vi "calibrationElectrometer_getEvent_settingsAppliedReadSets.vi"(8 "error in (no error)":errorcluster, 11 "logevent_settingsAppliedReadSets_Ctl":T1={"avgFilterType"=0, "electId"="                                                                                                                                                                                                                                                                ", "filterActive"=FALSE, "inputRange"=0.0, "integrationTime"=0.0, "medianFilterStatus"=FALSE, "mode"=0, "radingOption"=0, "readingTimeout"=0, "priority"=0}) -> (0 "error out":errorcluster, 2 "function return":i32, 3 "logevent_settingsAppliedReadSets_Ctl out":T1={"avgFilterType"=0, "electId"="                                                                                                                                                                                                                                                                ", "filterActive"=FALSE, "inputRange"=0.0, "integrationTime"=0.0, "medianFilterStatus"=FALSE, "mode"=0, "radingOption"=0, "readingTimeout"=0, "priority"=0})   [LabVIEW 2016, in "SALLV_calibrationElectrometer.lvlib"]
doc: "int calibrationElectrometer_shm_getEvent_settingsAppliedReadSetsLV(calibrationElectrometer_logevent_settingsAppliedReadSetsLV *logevent_settingsAppliedReadSets_Ctl );"
uses:
  SALLV_calibrationElectrometer.lvlib
  DataTypes/logevent_settingsAppliedReadSets.ctl
  SALLV_calibrationElectrometer.so
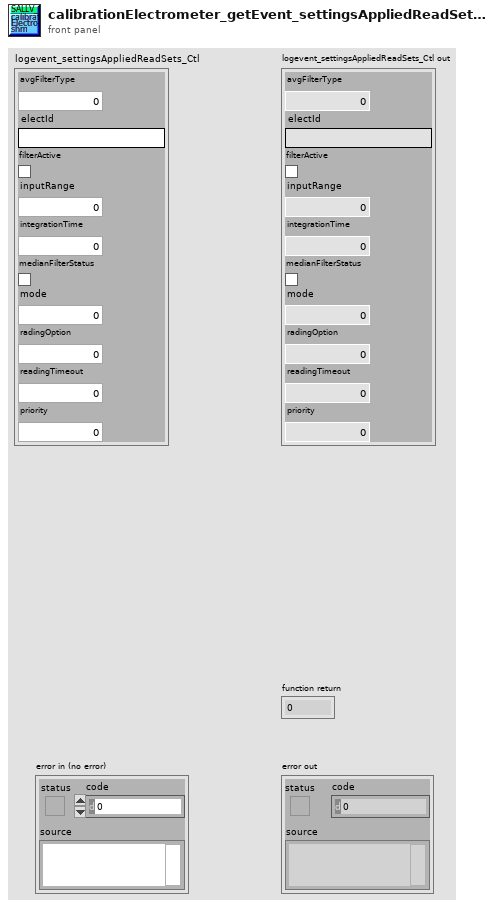
[diagram p1: front panel]
types:
  T1 = typedef "SALLV_calibrationElectrometer.lvlib/logevent_settingsAppliedReadSets.ctl" = cluster{"avgFilterType":i32, "electId":string, "filterActive":bool, "inputRange":dbl, "integrationTime":dbl, "medianFilterStatus":bool, "mode":i32, "radingOption":i32, "readingTimeout":i32, "priority":i32}
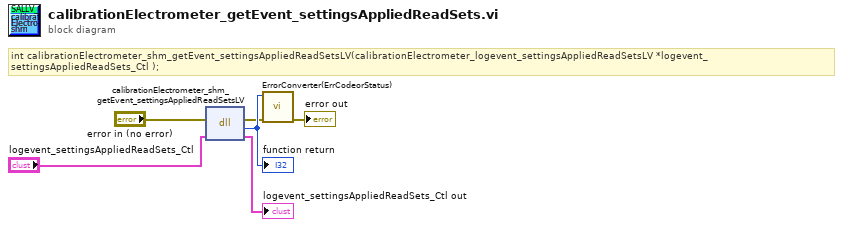
[diagram p0: block diagram]
diagram:
  # "int calibrationElectrometer_shm_getEvent_settingsAppliedReadSetsLV(calibrationElectrometer_logevent_settingsAppliedReadSetsLV *logevent_settingsAppliedReadSets_Ctl );"
  n1 = dll-call lib="home/andres/Desktop/SAL_calibrationElectrometer/SALLV_calibrationElectrometer.*" fn="calibrationElectrometer_shm_getEvent_settingsAppliedReadSetsLV"(error in="error in (no error)", "logevent_settingsAppliedReadSets_Ctl"="logevent_settingsAppliedReadSets_Ctl") -> (error out=w2:errorcluster, w6:i32, "logevent_settingsAppliedReadSets_Ctl"=→"logevent_settingsAppliedReadSets_Ctl out":T1)  [unwired: 2 in, 1 out]
  "function return" <- w6
  n2 = call "ErrorConverter(ErrCodeorStatus).vi"("error in (no error)"=w2, "error code"=w6) -> ("error out"=→"error out":errorcluster)  [unwired: 9 in]
